vi "LED trigger.vi"() -> ()   [LabVIEW 2012]
uses:
  <vilib>/DAQmx/create/channels.llb/DAQmx Create Channel (DO-Digital Output).vi
  <vilib>/DAQmx/write.llb/DAQmx Write (Digital Bool 1Line 1Point).vi
panel:
  out "error out":errorcluster
  in  "stop":bool
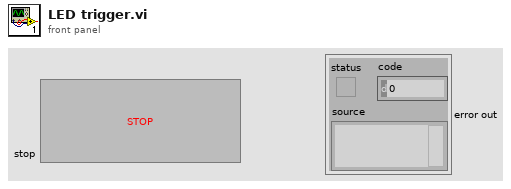
[diagram p1: front panel]
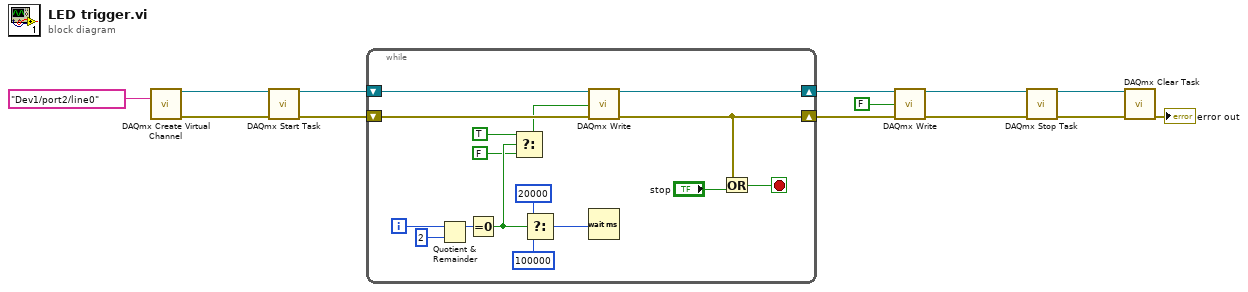
[diagram p0: block diagram]
diagram:
  n1 = call-poly <vilib>:"DAQmx Create Virtual Channel.vi"("lines"=tag "Dev1/port2/line0") -> ("task out"=w8:refnum<k21>, "error out"=w6:errorcluster)  [unwired: 13 in]
  n2 = call <vilib>:"DAQmx Start Task.vi"("task/channels in"=w8, "error in"=w6) -> ("task out"=w7:refnum<k21>, "error out"=w5:errorcluster)  [unwired: 12 in]
  n3 = while {
    shift-right: [w20] -> w12
    shift-left: w7 -> [w22]
    shift-right: [w16] -> w11
    shift-left: w5 -> [w21]
    i -> [w29]
    stop <- w14 stop-if-true
    n4 = Quotient & Remainder(x=w29, y=2) -> (x-y*floor(x/y)=w27:i32)  [unwired: 1 out]
    n5 = Equal To 0?(x=w27) -> (x = 0?=w26:bool)
    n6 = Select(t=TRUE, s=w26, f=FALSE) -> (s? t:f=w17:bool)
    n7 = Select(t=u32 20000 ("milliseconds to wait"), s=w26, f=u32 100000 ("milliseconds to wait")) -> (s? t:f=w23:u32)
    n8 = call-poly <vilib>:"DAQmx Write.vi"("task/channels in"=w22, "data"=w17, "error in"=w21) -> ("task out"=w20:refnum<k21>, "error out"=w16:errorcluster)  [unwired: 10 in, 1 out]
    n9 = Wait (ms)(milliseconds to wait=w23) -> ()  [unwired: 1 out]
    n10 = Or(x=w16, y="stop") -> (x .or. y?=w14:bool)
  }
  n11 = call-poly <vilib>:"DAQmx Write.vi"("task/channels in"=w12, "data"=FALSE, "error in"=w11) -> ("task out"=w2:refnum<k21>, "error out"=w4:errorcluster)  [unwired: 10 in, 1 out]
  n12 = call <vilib>:"DAQmx Stop Task.vi"("task/channels in"=w2, "error in"=w4) -> ("task out"=w1:refnum<k21>, "error out"=w3:errorcluster)  [unwired: 12 in]
  n13 = call <vilib>:"DAQmx Clear Task.vi"("task in"=w1, "error in"=w3) -> ("error out"=→"error out":errorcluster)  [unwired: 13 in]
